vi "MoveHUD.vi"(11 "VI":refnum<vi>) -> ()   [LabVIEW 2019]
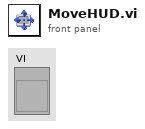
[diagram p1: front panel]
types:
  T1 = typedef "LVAllMonitorsDisplayTypeDef.ctl" = cluster{"Bounds":cluster{"Left":i16, "Top":i16, "Right":i16, "Bottom":i16}, "Depth":i16}[]
  T2 = cluster{"Left":i16, "Top":i16, "Right":i16, "Bottom":i16}
  T3 = cluster{"Bounds":cluster{"Left":i16, "Top":i16, "Right":i16, "Bottom":i16}, "Depth":i16}
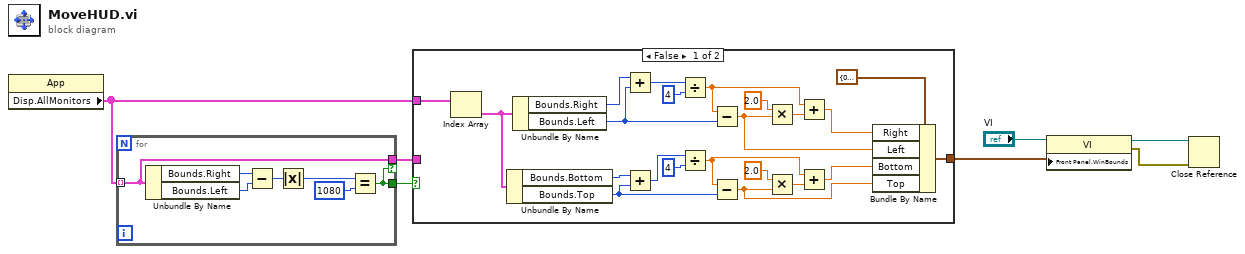
[diagram p0: block diagram]
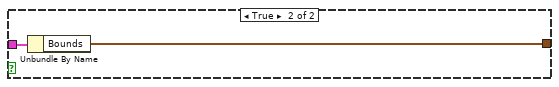
[diagram p2: hidden frame]
diagram:
  n1 = property class="App"() -> ("Disp.AllMonitors"=w2:T1)  [unwired: 2 in, 2 out]
  n2 = for {
    tunnel: w2 -> [w9] mode=indexing
    tunnel: [w8] -> w7
    tunnel: [w9] -> w6 if=w8
    n3 = Unbundle By Name(w9) -> ("Bounds.Right"=w13:i16, "Bounds.Left"=w14:i16)
    n4 = Subtract(x=w13, y=w14) -> (x-y=w12:i16)
    n5 = Absolute Value(x=w12) -> (abs(x)=w11:i16)
    n6 = Equal?(x=w11, y=i16 1080) -> (x = y?=w8:bool)
  }
  n7 = case shown="False" w7 {
    tunnel: w6 -> [_ w38]
    tunnel: [w32 w37] -> w5
    tunnel: w2 -> [w20 _]
    frame False {
      n8 = Index Array(array=w20) -> (element=w19:T3)  [unwired: 1 in]
      n9 = Unbundle By Name(w19) -> ("Bounds.Bottom"=w23:i16, "Bounds.Top"=w26:i16)
      n10 = Unbundle By Name(w19) -> ("Bounds.Right"=w36:i16, "Bounds.Left"=w31:i16)
      n11 = Add(x=w36, y=w31) -> (x+y=w35:i16)
      n12 = Add(x=w23, y=w26) -> (x+y=w24:i16)
      n13 = Divide(x=w35, y=i16 4) -> (x/y=w28:dbl)
      n14 = Divide(x=w24, y=i16 4) -> (x/y=w27:dbl)
      n15 = Subtract(x=w28, y=w31) -> (x-y=w29:dbl)
      n16 = Subtract(x=w27, y=w26) -> (x-y=w21:dbl)
      n17 = Multiply(x=2.0, y=w29) -> (x*y=w18:dbl)
      n18 = Multiply(x=2.0, y=w21) -> (x*y=w16:dbl)
      n19 = Add(x=w28, y=w18) -> (x+y=w30:dbl)
      n20 = Add(x=w27, y=w16) -> (x+y=w22:dbl)
      n21 = Bundle By Name(cluster=T2 {"Left"=0, "Top"=0, "Right"=0, "Bottom"=0} ("Bounds"), "Right"=w30, "Left"=w29, "Bottom"=w22, "Top"=w21) -> (w32:T2)
    }
    frame True {
      n22 = Unbundle By Name(w38) -> ("Bounds"=w37:T2)
    }
  }
  n23 = property class="VI"(reference="VI", "Front Panel.WinBounds"=w5) -> (reference out=w3:refnum<vi>, error out=w4:errorcluster)  [unwired: 1 in]
  n24 = Close Reference(reference=w3, error in (no error)=w4) -> ()  [unwired: 1 out]
